vi "load_adctest_descriptor_from_mat.vi"() -> ()   [LabVIEW 2012]
uses:
  <vilib>/imath/engines/lvmath/Functions/Error Handling/error.ctl
  <vilib>/imath/engines/lvmath2/RunTimeEngine/ErrorHandling/NIMS_Finalize Error.vi
  <vilib>/imath/engines/lvmath2/RunTimeEngine/Managers/WorkSpace/UID Generator.vi
  <vilib>/imath/engines/lvmath2/RunTimeEngine/NonStaticBuiltInFunctions/Manual/NIMS_NS_load.vi
  <vilib>/imath/engines/lvmath/Plug In/_Char/NIMS_CH_String to Character Array.vi
  <vilib>/imath/engines/lvmath2/RunTimeEngine/RunTimeType/NIMS_RunTimeType_From StrictType (excl LVString).vi
  <instcachedir>/0/NIMS_RunTimeType_From StrictType (excl LVString)_AC52D965D0864706932D20A05968E122.lvgen/NIMS_RunTimeType_From StrictType (excl LVString)_AC52D965D0864706932D20A05968E122_001.vi
  <vilib>/imath/engines/lvmath2/RunTimeEngine/Managers/SymbolTable/Write Variable.vi
  <vilib>/imath/engines/lvmath2/RunTimeEngine/RunTimeSymbolToken/NIMS_RunTimeSymbolToken_ReadVariable-1out.vi
  <vilib>/imath/engines/lvmath/Plug In/Control Design/RunTimeSymbolToken/NIMS_CD_RunTimeSymbolToken_ResolveSymbol.vi
  <instcachedir>/0/NIMS_CD_RunTimeSymbolToken_ResolveSymbol_821BF44DA7A542849A3EEBBC3B0CE636.lvgen/NIMS_CD_RunTimeSymbolToken_ResolveSymbol_821BF44DA7A542849A3EEBBC3B0CE636_001.vi
  <vilib>/imath/engines/lvmath2/RunTimeEngine/Struct/NIMS_NS_StructGetField.vi
  <vilib>/imath/engines/lvmath2/RunTimeEngine/LocalVariableDefStatement/MC_LocalVariableDefStatement_Display.vi
  <vilib>/imath/engines/lvmath2/RunTimeEngine/CommandStatement/NIMS_CommandStatement_MaskErr.vi
  <vilib>/imath/engines/lvmath2/RunTimeEngine/Managers/SymbolTable/Read Variable.vi
  <vilib>/imath/engines/lvmath2/RunTimeEngine/RunTimeType/NIMS_RunTimeType_Get Case Value.vi
  <vilib>/imathl/engines/lvmath/Functions/Error Handling/Create Error.vi
  <vilib>/imath/engines/lvmath/Functions/Error Handling/MergeErrorsWrapper.vi
  <vilib>/imath/engines/lvmath2/RunTimeEngine/NodeEndStatement/MC_NodeEndStatement_Dispose.vi
  <vilib>/imath/engines/lvmath2/RunTimeEngine/NodeEndStatement/NIMS_NodeEndStatement_Output.vi
  <instcachedir>/0/NIMS_NodeEndStatement_Output_53EC0D466D134D7ABD903AC30B43404B.lvgen/NIMS_NodeEndStatement_Output_53EC0D466D134D7ABD903AC30B43404B_005.vi
  <instcachedir>/0/NIMS_NodeEndStatement_Output_53EC0D466D134D7ABD903AC30B43404B.lvgen/NIMS_NodeEndStatement_Output_53EC0D466D134D7ABD903AC30B43404B_001.vi
  <instcachedir>/0/NIMS_NodeEndStatement_Output_53EC0D466D134D7ABD903AC30B43404B.lvgen/NIMS_NodeEndStatement_Output_53EC0D466D134D7ABD903AC30B43404B_013.vi
  <instcachedir>/0/NIMS_NodeEndStatement_Output_53EC0D466D134D7ABD903AC30B43404B.lvgen/NIMS_NodeEndStatement_Output_53EC0D466D134D7ABD903AC30B43404B_008.vi
  <instcachedir>/0/NIMS_NodeEndStatement_Output_53EC0D466D134D7ABD903AC30B43404B.lvgen/NIMS_NodeEndStatement_Output_53EC0D466D134D7ABD903AC30B43404B_009.vi
  <vilib>/imath/engines/lvmath/Plug In/Control Design/NonStaticBuiltInFunctions/NIMS_NS_is_field.vi
  <instcachedir>/0/NIMS_CD_RunTimeSymbolToken_ResolveSymbol_821BF44DA7A542849A3EEBBC3B0CE636.lvgen/NIMS_CD_RunTimeSymbolToken_ResolveSymbol_821BF44DA7A542849A3EEBBC3B0CE636_000.vi
  <vilib>/imath/engines/lvmath2/RunTimeEngine/IfStatement/NIMS_NS_IfCondition.vi
  <vilib>/imath/engines/lvmath/Plug In/Control Design/NonStaticBuiltInFunctions/NIMS_NS_ones.vi
  <instcachedir>/0/NIMS_RunTimeType_From StrictType (excl LVString)_AC52D965D0864706932D20A05968E122.lvgen/NIMS_RunTimeType_From StrictType (excl LVString)_AC52D965D0864706932D20A05968E122_000.vi
  <vilib>/imath/engines/lvmath/Plug In/Control Design/ArithmeticOperatorToken/NIMS_CD_NS_ArithmeticOperator_powermx.vi
  <vilib>/imath/engines/lvmath/Plug In/Control Design/ArithmeticOperatorToken/NIMS_CD_NS_ArithmeticOperator_minus.vi
  <vilib>/imath/engines/lvmath/Plug In/Control Design/ArithmeticOperatorToken/NIMS_CD_NS_ArithmeticOperator_multmx.vi
  <vilib>/imath/engines/lvmath2/RunTimeEngine/RunTimeType/NIMS_RunTimeType_To Numeric.vi
  <instcachedir>/0/NIMS_RunTimeType_To Numeric_F654E44AC9CD41E8ABC33AEB612B84CA.lvgen/NIMS_RunTimeType_To Numeric_F654E44AC9CD41E8ABC33AEB612B84CA_000.vi
  <vilib>/imath/engines/lvmath2/RunTimeEngine/NodeEndStatement/NIMS_NodeEndStatement_Get Scalar.vi
  <instcachedir>/0/NIMS_NodeEndStatement_Get Scalar_DDDE03B66C1B40AEB228387CE0451FA8.lvgen/NIMS_NodeEndStatement_Get Scalar_DDDE03B66C1B40AEB228387CE0451FA8_001.vi
  <vilib>/imath/engines/lvmath/Plug In/_Char/RunTimeType/NIMS_CH_RunTimeType_To Character 2D.vi
  <instcachedir>/0/NIMS_NodeEndStatement_Get Scalar_DDDE03B66C1B40AEB228387CE0451FA8.lvgen/NIMS_NodeEndStatement_Get Scalar_DDDE03B66C1B40AEB228387CE0451FA8_002.vi
  <vilib>/imath/engines/lvmath2/RunTimeEngine/NodeEndStatement/NIMS_NodeEndStatement_Get Vector.vi
  <instcachedir>/0/NIMS_NodeEndStatement_Get Vector_2BE3967F82A04EDB90B65AFAEF9E88C9.lvgen/NIMS_NodeEndStatement_Get Vector_2BE3967F82A04EDB90B65AFAEF9E88C9_002.vi
  <instcachedir>/0/NIMS_NodeEndStatement_Get Vector_2BE3967F82A04EDB90B65AFAEF9E88C9.lvgen/NIMS_NodeEndStatement_Get Vector_2BE3967F82A04EDB90B65AFAEF9E88C9_000.vi
  <vilib>/imath/engines/lvmath/Plug In/_Char/NIMS_CH_Character 1D to U8 1D.vi
  <vilib>/imath/engines/lvmath/Plug In/_Char/NIMS_CH_U8 2D to Character 2D.vi
  <vilib>/imath/engines/lvmath/Plug In/_Char/NIMS_CH_Character 2D to String 1D.vi
  <vilib>/imath/engines/lvmath/Plug In/_Char/NIMS_CH_U8 1D to Character 1D.vi
  <vilib>/imath/engines/lvmath/Plug In/_Char/NIMS_CH_Character RV to String.vi
  <vilib>/imath/engines/lvmath2/RunTimeEngine/Managers/SymbolTable/NIMS_WorkSpace.lvlib
panel:
  in  "Filename":path
  out "Comments on measurement":string[](array[string])
  out "Parameters: intergral nonlinearity (INL)":dbl[](array[numeric])
  out "Parameters: sigma (std. of noise on excitation signal)":dbl
  out "Parameters: theta (2*pi*f/fs)":dbl
  out "Parameters: C (DC component)":dbl
  out "Parameters: B (sine coeff)":dbl
  out "Parameters : A (cosine coeff)":dbl
  out "Simulated measurement":bool
  in  "Close":bool
  out "Measurement Record":dbl[](array[numeric])
  out "Number of Bits":dbl
  out "Channel":dbl
  out "Serial #":string
  out "Model":string
  out "Title of measurement":string
  in  "Load file":bool
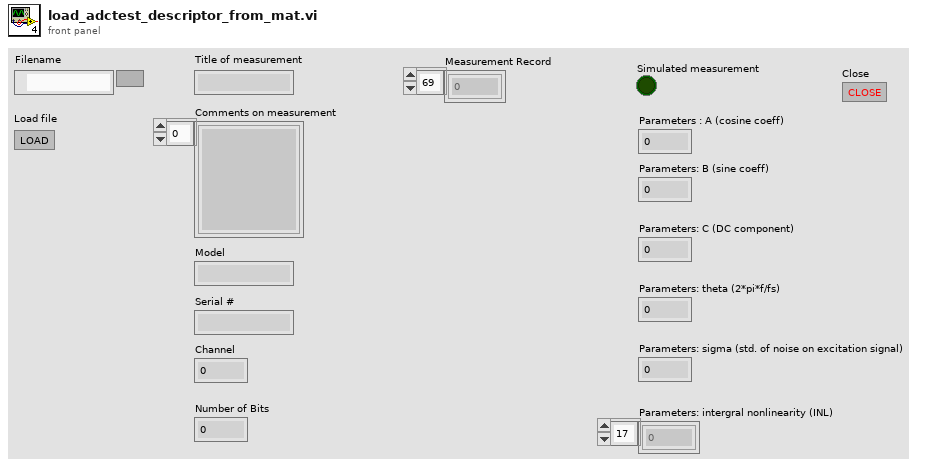
[diagram p1: front panel]
types:
  T1 = typedef "error.ctl" = enum16{"No Error", "Problem", "Input type must not be void", "Incorrect number of parameters", "Function not defined for non-numeric types", "An output variable of the user-defined function is undefined", "Function only defined for character arrays", "Function not defined for boolean, character, or single precision", "Function not defined for complex types", "Not a valid operation", "Inputs must be scalar", "Input matrices are not the same size", "Function only available on RT", "Input matrices must be nonnegative integers of the same type", "Arguments must be non-negative integers less than bitmax", "Number to complement must be less than 2^N", "Bit to get is outside range", "Bit to set is outside range", "Input must be real type ", "At least one parameter must be scalar", "Unable to display plug-in data on RT", "Function not defined for higher dimensional matrices", "Invalid attributes", "Wrong Type of Input Arguments", "Wrong Argument Option", "Invalid file identifier", "Indices must be real positive integers", "The variable is not a matrix data type.", "Number of elements must be the same for indices and values", "You cannot replace elements of a matrix with non-matrix data types.", "Cannot resize a 2D matrix with a linear index", "Unknown variable or symbol", "Indices out of range", "Empty matrix deletion can not be used with two indices", "Number of rows and columns must be the same for indices and values.", "Complex cannot be converted to Boolean", "Char cannot be converted to Boolean", "int64 cannot be converted to Boolean", "uint64 cannot be converted to Boolean", "You cannot convert a Boolean to a character.", "Incompatible input size in 3D surface function", "All rows must have the same number of columns", "Incompatible types", "Invalid matrix dimensions", "Dimension must be 1 or 2", "Base must be an integer between 2 and 36", "Invalid input", "Square matrix required", "Function 'timerstart' must be called before 'timerstop'", "Arguments must be positive real", "Step must not be zero", "Wrong number of input arguments", "Wrong number of output arguments", "Too many index arguments", "Input scalar must be >= 0", "Input scalar must be positive", "Input scalar must not be 0", "Input scalar must be in range [0,1]", "Can't use conditionally defined variable that's undefined", "Input must be a vector", "RT Exec Trace Toolkit not licensed", "Empty vector error", "All elements must be in domain [-1,1]", "All real elements of input vector must be >= 0", "All elements of input vector must be positive", "Values of input vectors are not compatible", "DAQmx not installed", "Input vector must be an increasing vector", "Dereferenced field does not exist within the struct", "A vector or matrix of structures must be indexed before it can be dereferenced", "Lenths of two input vectors are not compatible", "Invalid fieldname", "Empty matrix error", "Cannot use '.' on a type other than Struct", "Unused074", "Data type of the struct's field name is invalid", "Using . to dereference data that is not a struct", "Input struct contains invalid type ", "Size of input matrix is incompatible with input size", "Invalid format specifier", "Could not find field within struct", "Bad permutation array", "Mismatched fieldnames", "ode: User Function could not be opened", "ode: User Function signature does not meet ode requirements", "Unused085", "RunTime: MathScript could not be compiled", "Unknown function", "Only scalars and strings supported", "ode: User Function signature has incorrect number of inputs", "ode:User Function signature has incorrect number of outputs", "Range is too large", "End used without variable", "Function not available (RTE)", "Custom user error", "Arguments must be integers less than bitmax", "Shared library not found", "Header file not found", "Shared library already loaded", "Shared library not loaded", "Shared library function not found", "Shared library string return problem", "Problem calling shared library function", "Problem loading shared library from OS", "Problem parsing shared library header file", "Shared library incompatible types", "Shared library unsupported return type", "Shared library function not exported", "Shared library unsupported input type", "Problem unloading shared library from OS", "Function only available from UI", "Function specified in argument is missing", "An internal error has occurred", "Invalid object", "Invalid property", "Read-only property", "A break command has occurred", "A continue command has occurred", "A return command has occurred", "ode: times parameter invalid", "Function specified in argument has incorrect signature", "Function not found in file", "Reserved keyword cannot be defined as variable", "Reserved keyword cannot be defined as a function or script", "Arguments must be string literals", "Function not supported on this platform", "All columns must have the same number of rows", "Function ignored in RTE warning", "Cannot use : as a parameter that is not a variable", "Output can't be coerced to requested type", "Function not supported on current target", "Variable dependent on an unwired function input", "Unused132", "Unused133", "Unused134", "Unused135", "Unused136", "Unused137", "Unused138", "Unused139", "Unused140", "Unused141", "Unused142", "Invalid output type. Cannot output a cell array of any type other than string.", "Invalid output type. Type is a dynamic struct.", "Invalid output type. Type is a struct that has a field whose type is not known until run-time", "Invalid output type. Type is a struct that has a field which is a plot object.", "MathScript parser DLL missing", "MathScript requires LabVIEW Full", "MathScript license is invalid or missing"}
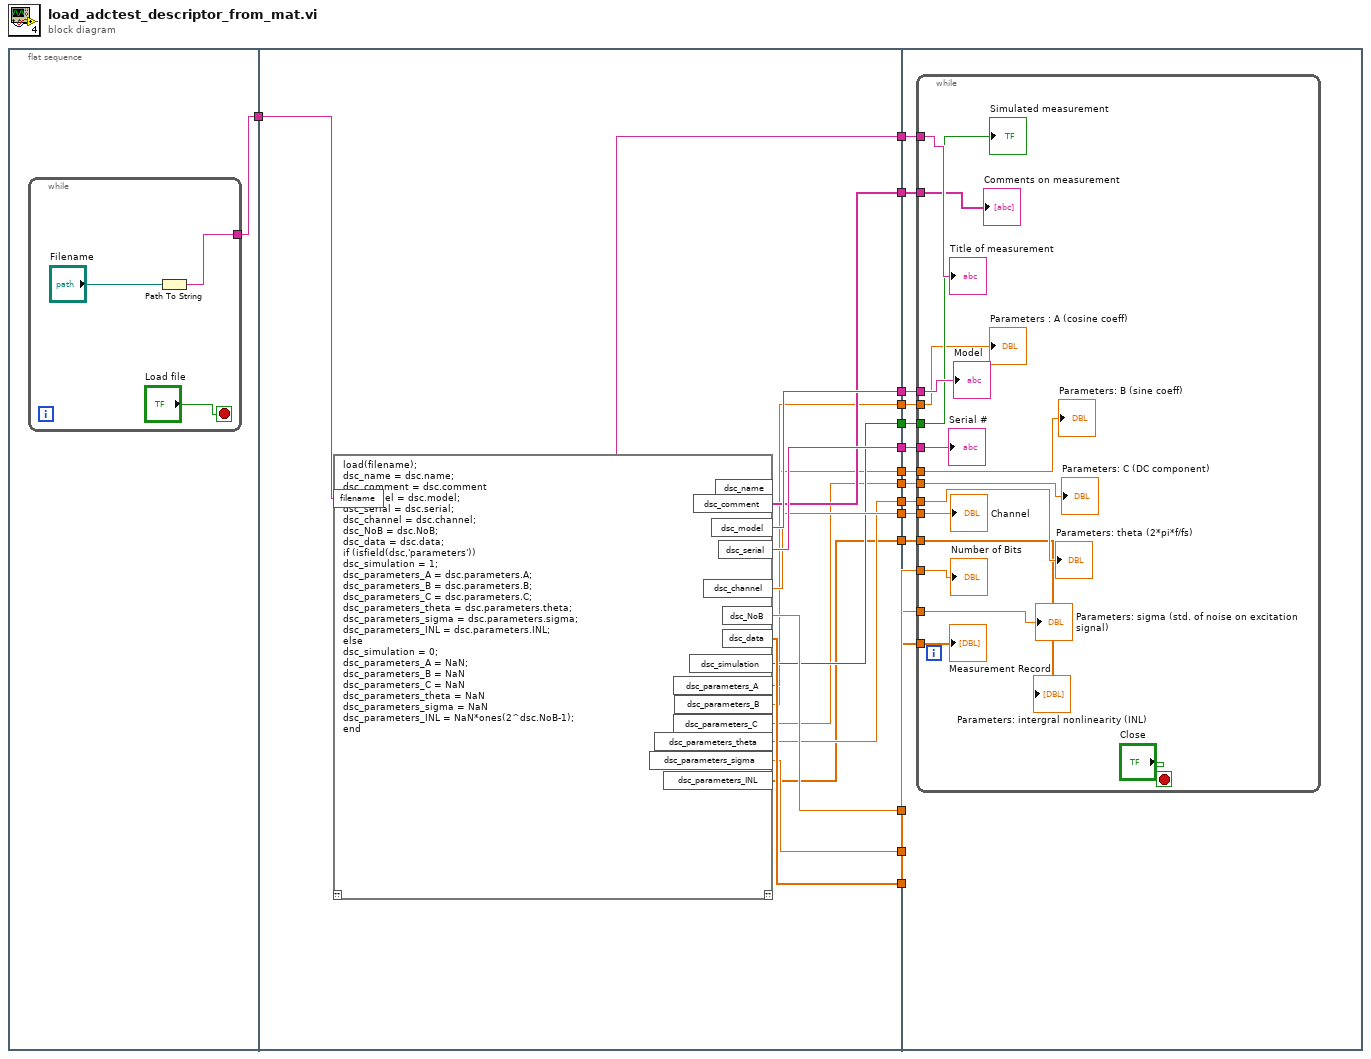
[diagram p0: block diagram]
diagram:
  n1 = flat-sequence {
    tunnel: [w16] -> w15
    tunnel: w15 -> [w34]
    tunnel: [w33] -> w14
    tunnel: [w32] -> w13
    tunnel: [w31] -> w12
    tunnel: [w30] -> w11
    tunnel: [w29] -> w10
    tunnel: [w28] -> w9
    tunnel: [w27] -> w8
    tunnel: [w26] -> w7
    tunnel: [w25] -> w6
    tunnel: [w24] -> w5
    tunnel: [w23] -> w4
    tunnel: [w22] -> w3
    tunnel: [w21] -> w2
    tunnel: [w20] -> w1
    tunnel: w14 -> [w1130]
    tunnel: w13 -> [w1129]
    tunnel: w12 -> [w1128]
    tunnel: w11 -> [w1127]
    tunnel: w10 -> [w1126]
    tunnel: w9 -> [w1125]
    tunnel: w8 -> [w1124]
    tunnel: w7 -> [w1123]
    tunnel: w6 -> [w1122]
    tunnel: w5 -> [w1121]
    tunnel: w4 -> [w1120]
    tunnel: w3 -> [w1119]
    tunnel: w2 -> [w1118]
    tunnel: w1 -> [w1117]
    frame #0 {
      n2 = while {
        tunnel: [w17] -> w16
        stop <- "Load file" stop-if-true
        n3 = Path To String(path="Filename") -> (string=w17:string)
      }
    }
    frame #1 {
      n4 = mathscript code="load(filename);\ndsc_name = dsc.name;\ndsc_comment = dsc.comment\ndsc_model = dsc.model;\ndsc_serial = dsc.serial;\ndsc_channel = dsc.channel;\ndsc_NoB = dsc.NoB;\ndsc_data = dsc.data;\nif (isfield(dsc,'parameters'))\ndsc_simulation = 1;\ndsc_parameters_A = dsc.parameters.A;\ndsc_parameters_B = dsc.parameters.B;\ndsc_parameters_C = dsc.parameters.C;\ndsc_parameters_theta = dsc.parameters.theta;\ndsc_parameters_sigma = dsc.parameters.sigma;\ndsc_parameters_INL = dsc.parameters.INL;\nelse\ndsc_simulation = 0;\ndsc_parameters_A = NaN;\ndsc_parameters_B = NaN\ndsc_parameters_C = NaN\ndsc_parameters_theta = NaN\ndsc_parameters_sigma = NaN\ndsc_parameters_INL = NaN*ones(2^dsc.NoB-1);\nend"("filename"=w34) -> ("dsc_name"=w33:string, "dsc_model"=w32:string, "dsc_serial"=w31:string, "dsc_channel"=w30:dbl, "dsc_NoB"=w29:dbl, "dsc_data"=w28:dbl[], "dsc_comment"=w27:string[], "dsc_simulation"=w26:bool, "dsc_parameters_A"=w25:dbl, "dsc_parameters_B"=w24:dbl, "dsc_parameters_C"=w23:dbl, "dsc_parameters_theta"=w22:dbl, "dsc_parameters_sigma"=w21:dbl, "dsc_parameters_INL"=w20:dbl[])  [unwired: 1 in, 1 out]
    }
    frame #2 {
      n5 = while {
        tunnel: w1130 -> [w1145]
        tunnel: w1129 -> [w1144]
        tunnel: w1128 -> [w1143]
        tunnel: w1127 -> [w1142]
        tunnel: w1126 -> [w1141]
        tunnel: w1125 -> [w1140]
        tunnel: w1124 -> [w1131]
        tunnel: w1123 -> [w1138]
        tunnel: w1122 -> [w1137]
        tunnel: w1121 -> [w1136]
        tunnel: w1120 -> [w1135]
        tunnel: w1119 -> [w1134]
        tunnel: w1118 -> [w1133]
        tunnel: w1117 -> [w1132]
        stop <- "Close" stop-if-true
        "Title of measurement" <- w1145
        "Model" <- w1144
        "Serial #" <- w1143
        "Channel" <- w1142
        "Number of Bits" <- w1141
        "Measurement Record" <- w1140
        "Simulated measurement" <- w1138
        "Parameters : A (cosine coeff)" <- w1137
        "Parameters: B (sine coeff)" <- w1136
        "Parameters: C (DC component)" <- w1135
        "Parameters: theta (2*pi*f/fs)" <- w1134
        "Parameters: sigma (std. of noise on excitation signal)" <- w1133
        "Parameters: intergral nonlinearity (INL)" <- w1132
        "Comments on measurement" <- w1131
      }
    }
  }
